vi "Load Xml(traverse).vi"(8 "error in":errorcluster caption="错误输入（无错误）", 10 "Data in":T1, 11 "PanelRootNode.lvclass":refnum<class "PanelRootNode.lvclass">) -> (0 "error out":errorcluster caption="错误输出", 2 "DOM Ref":refnum<k20>, 3 "PanelRootNode out":refnum<class "PanelRootNode.lvclass">)   [LabVIEW 2016, in "PanelRootNode.lvclass"]
uses:
  PanelRootNode.lvclass
  C:/Users/CL/Desktop/ZcDAQprj0811/ZcDAQprj/Modules/DAQ-Display/PanelSplitToolkit/PanelLinkNode/PanelLinkNode.lvclass
  PanelLinkNode/PanelLinkNode.lvclass/PanelLinkNode.ctl
  PanelObject/PanelObject.lvclass
  PanelLinkNode/PanelLinkNode.lvclass
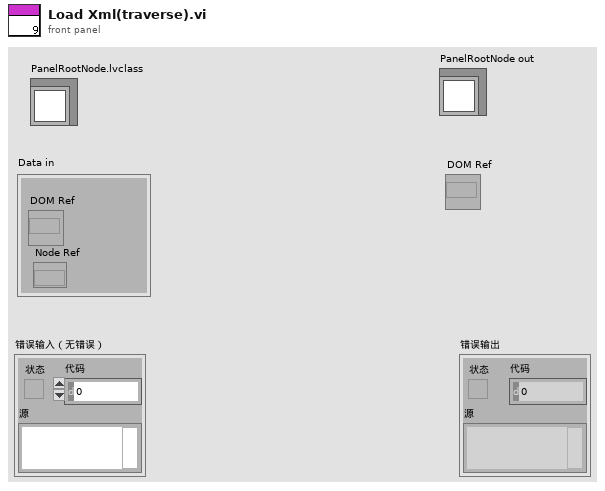
[diagram p1: front panel]
types:
  T1 = cluster{"DOM Ref":refnum<k20>, "Node Ref":refnum<k20>}
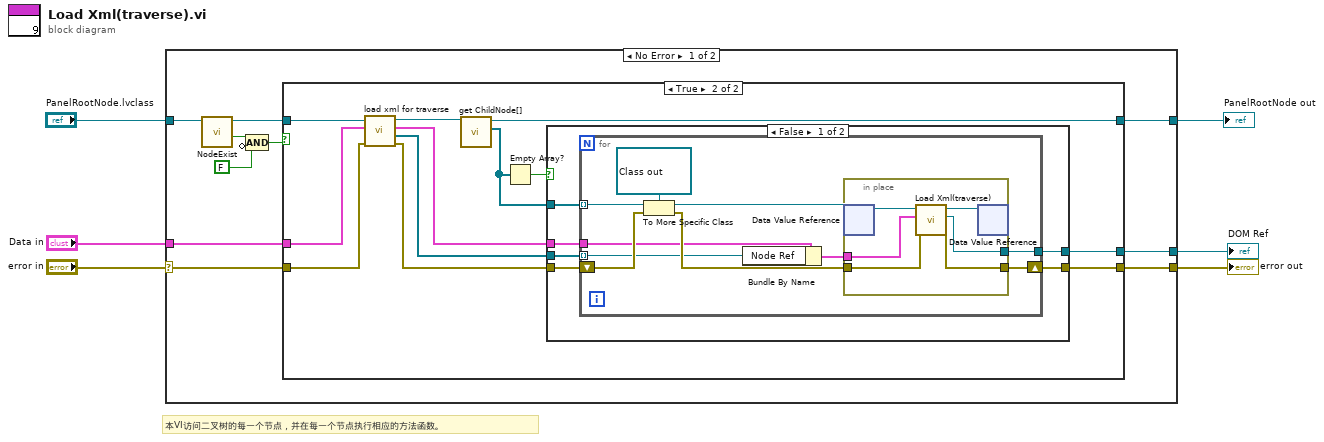
[diagram p0: block diagram]
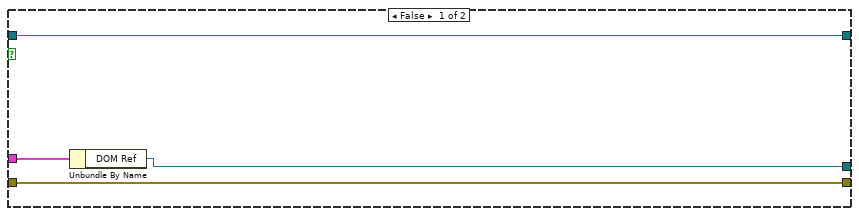
[diagram p2: hidden frame]
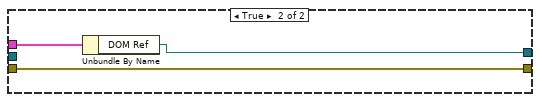
[diagram p3: hidden frame]
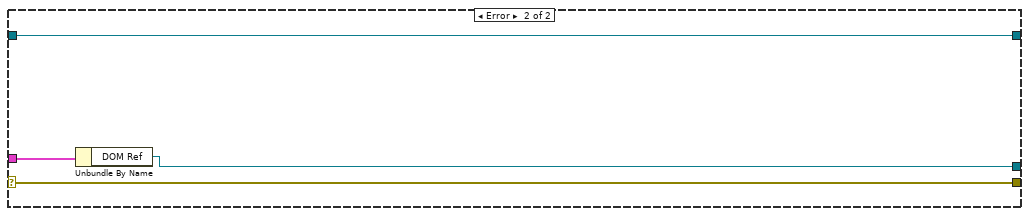
[diagram p4: hidden frame]
diagram:
  # "本VI访问二叉树的每一个节点，并在每一个节点执行相应的方法函数。"
  n1 = case shown="No Error" "error in" {
    selector: "error in" -> [w10 w61]
    tunnel: [w13 w61] -> w5
    tunnel: [w16 w60] -> w3
    tunnel: "PanelRootNode.lvclass" -> [w15 w60]
    tunnel: "Data in" -> [w8 w59]
    tunnel: [w7 w58] -> w1
    frame No Error {
      n2 = call-dynamic "NodeExist.vi"("PanelLinkNode 输入"=w15) -> ("Node Exist?"=w12:bool, "PanelLinkNode 输出"=w14:refnum<class "PanelRootNode.lvclass">)  [unwired: 8 in, 1 out]
      n3 = Compound Arithmetic op=AND(w12, invert FALSE ("值")) -> (w11:bool)
      n4 = case shown="True" w11 {
        tunnel: [w20 w32] -> w16
        tunnel: w14 -> [w20 w29]
        tunnel: [w19 w22] -> w13
        tunnel: w10 -> [w19 w26]
        tunnel: w8 -> [w18 w27]
        tunnel: [w17 w21] -> w7
        frame False {
          n5 = Unbundle By Name(w18) -> ("DOM Ref"=w17:refnum<k20>)
        }
        frame True {
          n6 = call "load xml for traverse.vi"("error in"=w26, "Data in"=w27, "PanelRootNode 输入"=w29) -> ("error out"=w24:errorcluster, "SubNodes"=w23:refnum<k20>[], "Data out"=w25:T1, "PanelRootNode 输出"=w28:refnum<class "PanelRootNode.lvclass">)  [unwired: 5 in]
          n7 = call "get ChildNode[].vi"("PanelLinkNode输入"=w28) -> ("ChildNode*[]"=w31:refnum<data-value>[], "PanelLinkNode输出"=w32:refnum<class "PanelRootNode.lvclass">)  [unwired: 8 in, 1 out]
          n8 = Empty Array?(array=w31) -> (empty?=w30:bool)
          n9 = case shown="False" w30 {
            tunnel: w31 -> [w38 _]
            tunnel: [w37 w57] -> w22
            tunnel: w25 -> [w36 w56]
            tunnel: w24 -> [w35 w57]
            tunnel: w23 -> [w34 _]
            tunnel: [w33 w55] -> w21
            frame False {
              n10 = for {
                tunnel: w38 -> [w48] mode=indexing
                shift-right: [w43] -> w37
                shift-left: w35 -> [w46]
                tunnel: w36 -> [w41]
                tunnel: w34 -> [w42] mode=indexing
                tunnel: [w39] -> w33
                n11 = To More Specific Class(target class=refnum<data-value> refnum ("数据值引用"), reference=w48, error in=w46) -> (specific class reference=w47:refnum<data-value>, error out=w45:errorcluster)
                n12 = Bundle By Name(cluster=w41, "Node Ref"=w42) -> (w40:T1)
                n13 = in-place {
                  in-place-border: w45 -> [w51]
                  in-place-border: w40 -> [w52]
                  in-place-border: [w50] -> w43
                  in-place-border: [w49] -> w39
                  n14 = in-place-dvr #1(w47) -> (w54:refnum<class "PanelRootNode.lvclass">)  [unwired: 1 out]
                  n15 = call "Load Xml(traverse).vi"("error in"=w51, "Data in"=w52, "PanelRootNode.lvclass"=w54) -> ("error out"=w50:errorcluster, "DOM Ref"=w49:refnum<k20>, "PanelRootNode out"=w53:refnum<class "PanelRootNode.lvclass">)  [unwired: 6 in]
                  n16 = in-place-dvr #1(w53) -> ()  [unwired: 2 out]
                }
              }
            }
            frame True {
              n17 = Unbundle By Name(w56) -> ("DOM Ref"=w55:refnum<k20>)
            }
          }
        }
      }
    }
    frame Error {
      n18 = Unbundle By Name(w59) -> ("DOM Ref"=w58:refnum<k20>)
    }
  }
  "error out" <- w5
  "PanelRootNode out" <- w3
  "DOM Ref" <- w1
